vi "GetParam.vi"(8 "error in (no error)":errorcluster caption="entrée d'erreur (pas d'erreur)", 11 "KBinsDiscretizer.lvclass":refnum<class "KBinsDiscretizer.lvclass">) -> (0 "error out":errorcluster caption="sortie d'erreur", 2 "KBinsDiscretizer":T1={"n_bins"=[5], "encode"="onehot", "strategy"="quantile"}, 3 "KBinsDiscretizer.lvclass":refnum<class "KBinsDiscretizer.lvclass">)   [LabVIEW 2020, in "KBinsDiscretizer.lvclass"]
doc: "Get Parameters"
uses:
  KBinsDiscretizer.lvclass
  KBinsDiscretizer.lvclass/KBinsDiscretizer.ctl
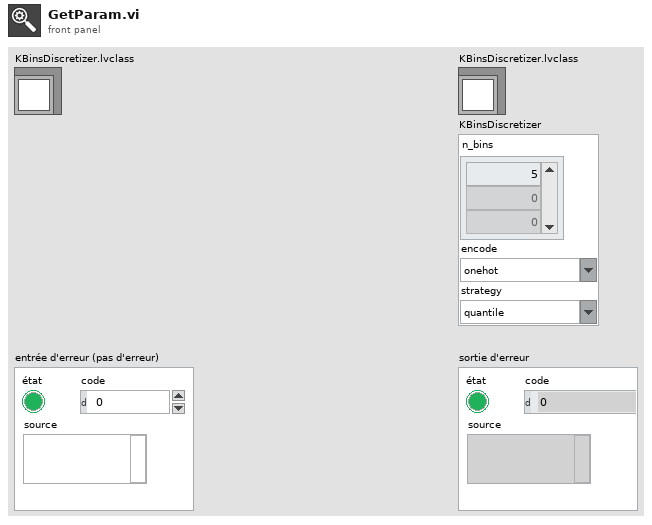
[diagram p1: front panel]
types:
  T1 = cluster{"n_bins":i32[], "encode":string, "strategy":string}
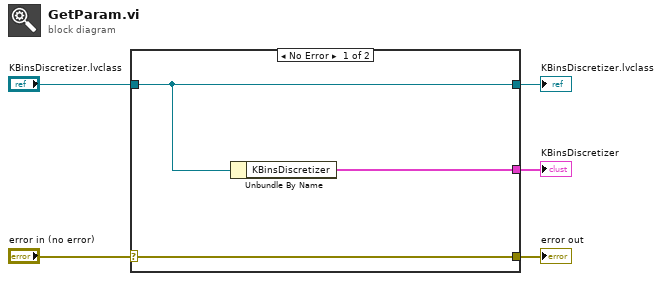
[diagram p0: block diagram]
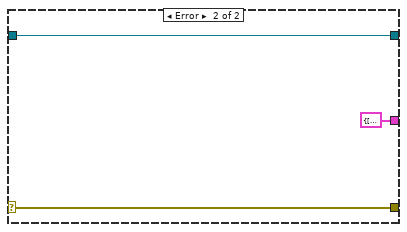
[diagram p2: hidden frame]
diagram:
  n1 = case shown="No Error" "error in (no error)" {
    selector: "error in (no error)" -> [w8 w10]
    tunnel: [w8 w10] -> w4
    tunnel: [w7 w11] -> w2
    tunnel: "KBinsDiscretizer.lvclass" -> [w7 w11]
    tunnel: [w6 T1 {"n_bins"=[], "encode"="", "strategy"=""} ("KBinsDiscretizer")] -> w1
    frame No Error {
      n2 = Unbundle By Name(w7) -> ("KBinsDiscretizer"=w6:T1)
    }
    frame Error {
    }
  }
  "error out" <- w4
  "KBinsDiscretizer.lvclass" <- w2
  "KBinsDiscretizer" <- w1
